vi "2_Sin(x)_Cos(x)(Inference).vi"() -> ()   [LabVIEW 2020]
uses:
  <vilib>/Ngene/DeepLTK/Toolkit/NN_Network/Controls/NN_Save_Before_Destroy_Options.ctl
  <vilib>/Ngene/DeepLTK/Toolkit/NN_Layers/Layers/Input/API/NN_Layer_Set_Out(Input1D_idx).vi
  <vilib>/Ngene/DeepLTK/Toolkit/Deep_Learning_Toolkit_by_Ngene.lvlib
panel:
  out "Absalut Error Precentage cos(x)":sgl=0.004982114 format="%#_2g%%"
  out "Absalut Error Precentage sin(x)":sgl=0.004982114 format="%#_2g%%"
  out "cos(x) Ground Truth":sgl=0.44851217
  out "cos(x) Predicted":sgl=0.44892797
  out "sin(x) Predicted":sgl=-0.89715314
  out "sin(x) Ground Truth":sgl=-0.8937767
  in  "Stop":bool
  in  "Weight File Path":path=path "D:/Ngene/Projects_SVN/DeepLTK/Examples/1_Simple_Examples/15_Multiple_output_regression_Sin(x)_Cos(x)/working/Sin(x)_Cos(x)/Sin(x)_Cos(x)_weights_23_08_02__16_20_12.bin"
  in  "CFG File Path":path=path "D:/Ngene/Projects_SVN/DeepLTK/Examples/1_Simple_Examples/15_Multiple_output_regression_Sin(x)_Cos(x)/working/Sin(x)_Cos(x)/Sin(x)_Cos(x)_net_cfg_23_08_02__16_20_12.cfg"
  in  "Input (radians)":sgl(slide)=11.460674 scale=0.0..30.0
  # "Overview: Demonstrates the usage of DeepLTK(Deep Learning Toolkit for LabVIEW) for solving a simple regression problem of modeling sin(x) and cos(x) functions\nRequirements: DeepLTK - Deep Learning Toolkit for LabVIEW (https://www.ngene.co/deep-learning-toolkit-for-labview)\n\nInstructions:\n1. Provide Network Configuration File Path and Weight File Path generated from \"1_Sin(x)_Cos(x)(Training).vi\".\n2. Run the VI.\n3. Provide input values at Input (radians) control and observe predicted values for sin(x) at sin(x) Predicted and compare it with sin(x) Ground Truth and same with cos(x). \n4. Press the Stop button to stop the VI.\n\nMore Examples:  https://github.com/ngenehub/deepltk_examples"
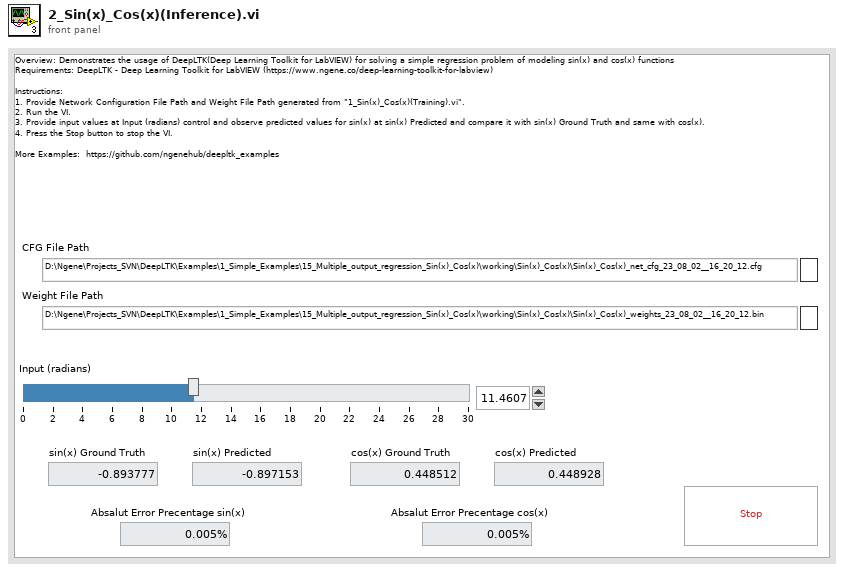
[diagram p1: front panel]
types:
  T1 = typedef "Deep_Learning_Toolkit_by_Ngene.lvlib/NN_Save_Before_Destroy_Options.ctl" = cluster{"CFG?":bool, "Weights?":bool, "Render?":bool}
  T2 = typedef "Deep_Learning_Toolkit_by_Ngene.lvlib/NN_Config_Params.ctl" = cluster{"Name":string, "mBatch":i32, "NN_Train_Params":T3, "LR_Decay_Policy":T6, "Labels":string[], "Loss":T8}
  T3 = typedef "Deep_Learning_Toolkit_by_Ngene.lvlib/NN_Train_Params.ctl" = cluster{"Optimizer":T4, "Beta_1":sgl, "Beta_2":sgl, "Weight Decay(L1)":sgl, "Weight Decay(L2)":sgl, "Data_Sampling":T5}
  T4 = typedef "Deep_Learning_Toolkit_by_Ngene.lvlib/NN_Train_Optimizer.ctl" = enum16{"SGD", "Adam", "Adagrad", "Adadelta", "RMSProp", "Nesterov"}
  T5 = typedef "Deep_Learning_Toolkit_by_Ngene.lvlib/NN_Train_Data_Sampling.ctl" = enum16{"Random", "Sequential"}
  T6 = typedef "Deep_Learning_Toolkit_by_Ngene.lvlib/NN_LR_Policy_Cfg.ctl" = cluster{"Policy_Type":T7, "LR0":dbl, "k":sgl, "WarmUp_Policy":enum16{"Step", "Ramp"}, "WarmUp_Iter":i32, "WarmUp_Ratio":sgl}
  T7 = typedef "Deep_Learning_Toolkit_by_Ngene.lvlib/NN_LR_Policy_Type.ctl" = enum16{"Manual", "Step", "Exp", "1/t"}
  T8 = typedef "Deep_Learning_Toolkit_by_Ngene.lvlib/NN_Loss_Config_Params.ctl" = cluster{"Loss_Type":T9, "Loss_Conf_Params":variant}
  T9 = typedef "Deep_Learning_Toolkit_by_Ngene.lvlib/NN_Loss_Type.ctl" = enum16{"None", "MSE", "CrossEntropy", "YOLO_v2"}
  T10 = typedef "Deep_Learning_Toolkit_by_Ngene.lvlib/NN_Layer_Config_Params.ctl" = cluster{"Layer_Type":T11, "Layer_Conf_Params":variant}
  T11 = typedef "Deep_Learning_Toolkit_by_Ngene.lvlib/NN_Layer_Type.ctl" = enum16{"Input1D", "Input3D", "Conv2D", "Conv2D_Adv", "MaxPool", "AvgPool", "UpSample", "DropOut3D", "ShortCut", "Concat", "SoftMax3D", "FC", "DropOut", "Softmax", "Flatten", "YOLO_v2", "Unsupported"}
  T12 = typedef "Deep_Learning_Toolkit_by_Ngene.lvlib/NN.ctl" = cluster{"Name":string, "No of Layers":i32, "mBatch":i32, "Layers":T13[], "Dimty":T14, "Dims_In":T15, "Dims_Out":T15, "Working_Dir":path, "Train?":bool, "Train_Params":T3, "LR_Update_Policy":T6, "Session Data":T16, "Ground_truth":T17, "NNg_hdls":T19, "NN_Device":T20, "GPU Id":i32, "Labels":string[], "Receptive Field":T21[], "Loss_Type":T9, "Loss_Cfg_Prms":variant}
  T13 = typedef "Deep_Learning_Toolkit_by_Ngene.lvlib/NN_Layer_ref.ctl" = refnum<data-value>
  T14 = typedef "Deep_Learning_Toolkit_by_Ngene.lvlib/NN_In_Out_Dim-ty.ctl" = enum8{"In1D_Out1D", "In3D_Out1D", "In3D_Out3D", "In3D_OutBBox"}
  T15 = typedef "Deep_Learning_Toolkit_by_Ngene.lvlib/NN_Dims(C,H,W).ctl" = cluster{"C":i32, "H":i32, "W":i32}
  T16 = typedef "Deep_Learning_Toolkit_by_Ngene.lvlib/NN_Train_Session_Data.ctl" = cluster{"Epochs":sgl, "Tot_Iter":i32, "LR":sgl, "LR_iter":i32}
  T17 = typedef "Deep_Learning_Toolkit_by_Ngene.lvlib/NN_Ground_truth.ctl" = cluster{"Y":variant, "Y_idx":T18}
  T18 = typedef "Deep_Learning_Toolkit_by_Ngene.lvlib/NN_Data_ref(1D_I32).ctl" = refnum<data-value>
  T19 = typedef "Deep_Learning_Toolkit_by_Ngene.lvlib/nng_cuda_handles.ctl" = cluster{"cudnn":u64, "cublas":u64, "stream":u64, "curand":u64}
  T20 = typedef "Deep_Learning_Toolkit_by_Ngene.lvlib/NN_Device.ctl" = enum16{"CPU", "GPU"}
  T21 = typedef "Deep_Learning_Toolkit_by_Ngene.lvlib/NN_Dims(V,H).ctl" = cluster{"V":i32, "H":i32}
  T22 = typedef "Deep_Learning_Toolkit_by_Ngene.lvlib/NN_Layer.ctl" = cluster{"Name":string, "Layer_Data":variant, "Layer_Type":T11, "Dims_In":T15, "Layers_In":variant, "Dims_Out":T15, "Layers_Out":variant, "Metrics":T23, "GPU_Data":variant, "mBatch":i32, "NN_Device":T20, "NNg_hdls":T19, "Train?":bool, "Dimty":T24, "RecptField":T25}
  T23 = typedef "Deep_Learning_Toolkit_by_Ngene.lvlib/NN_Layer_Metrics.ctl" = cluster{"Data":dbl, "Params":dbl, "Ops":dbl}
  T24 = typedef "Deep_Learning_Toolkit_by_Ngene.lvlib/NN_Layer_Dimty.ctl" = enum16{"1D", "3D"}
  T25 = typedef "Deep_Learning_Toolkit_by_Ngene.lvlib/NN_Layer_RF_State.ctl" = cluster{"Dims":T21, "J":T21}
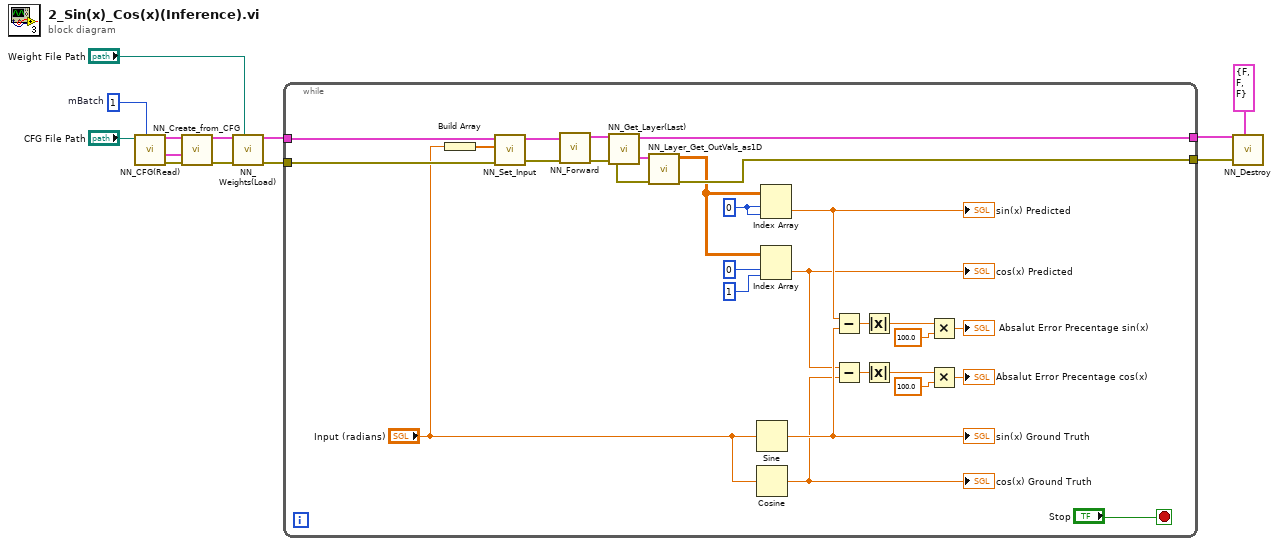
[diagram p0: block diagram]
diagram:
  w4 = 1  # mBatch
  n1 = call <vilib>:"NN_CFG(Read).vi"("mBatch"=w4, "CFG file path"="CFG File Path") -> ("error out"=w13:errorcluster, "Net_Cfg"=w5:T2, "Layer_Cfg"=w10:T10[])  [unwired: 7 in]
  n2 = call <vilib>:"NN_Create_from_CFG.vi"("error in (no error)"=w13, "Net_Cfg"=w5, "Layer_Cfg"=w10) -> ("error out"=w12:errorcluster, "NN out"=w11:T12)  [unwired: 7 in]
  n3 = call <vilib>:"NN_Weights(Load).vi"("Weight File Path"="Weight File Path", "error in (no error)"=w12, "NN in"=w11) -> ("error out"=w8:errorcluster, "NN out"=w9:T12)  [unwired: 7 in]
  n4 = while {
    tunnel: w9 -> [w41]
    tunnel: w8 -> [w42]
    tunnel: [w34] -> w7
    tunnel: [w31] -> w6
    stop <- "Stop" stop-if-true
    w33 = 0 ("disabled index (col)")
    n5 = Build Array("Input (radians)") -> (w32:sgl[])
    n6 = call-poly <vilib>:"NN_Set_Input.vi"("error in (no error)"=w42, "Data_In(1D_SGL)"=w32, "NN In"=w41) -> ("error out"=w39:errorcluster, "NN Out"=w40:T12)  [unwired: 7 in]
    n7 = call <vilib>:"NN_Forward.vi"("error in (no error)"=w39, "NN in"=w40) -> ("error out"=w38:errorcluster, "NN out"=w37:T12)  [unwired: 6 in, 2 out]
    n8 = call <vilib>:"NN_Get_Layer(Last).vi"("error in (no error)"=w38, "NN in"=w37) -> ("error out"=w36:errorcluster, "Last_Layer"=w35:T22, "NN out"=w34:T12)  [unwired: 6 in, 1 out]
    n9 = call <vilib>:"NN_Layer_Get_OutVals_as1D.vi"("error in (no error)"=w36, "Layer"=w35) -> ("error out"=w31:errorcluster, "Out(as1D)"=w28:sgl[][])  [unwired: 8 in]
    n10 = Sine(x="Input (radians)") -> (sin(x)=w21:sgl)
    "sin(x) Ground Truth" <- w21
    n11 = Cosine(x="Input (radians)") -> (cos(x)=w14:sgl)
    "cos(x) Ground Truth" <- w14
    n12 = Index Array(array=w28, index (row)=w33, index (col)=w33) -> (element=w20:sgl)
    "sin(x) Predicted" <- w20
    n13 = Index Array(array=w28, index (row)=0 ("disabled index (col)"), index (col)=1 ("disabled index (col)")) -> (element=w15:sgl)
    "cos(x) Predicted" <- w15
    n14 = Subtract(x=w20, y=w21) -> (x-y=w25:sgl)
    n15 = Subtract(x=w15, y=w14) -> (x-y=w19:sgl)
    n16 = Absolute Value(x=w25) -> (abs(x)=w24:sgl)
    n17 = Absolute Value(x=w19) -> (abs(x)=w18:sgl)
    n18 = Multiply(x=w24, y=sgl 100.0) -> (x*y=→"Absalut Error Precentage sin(x)":sgl)
    n19 = Multiply(x=w18, y=sgl 100.0) -> (x*y=→"Absalut Error Precentage cos(x)":sgl)
  }
  n20 = call <vilib>:"NN_Destroy.vi"("Save (T, T, T)"=T1 {"CFG?"=FALSE, "Weights?"=FALSE, "Render?"=FALSE}, "error in (no error)"=w6, "NN in"=w7) -> ()  [unwired: 8 in, 1 out]
